vi "PvgeneratorOP300.vi"(8 "errin":errorcluster, 9 "BDD 2":T1, 10 "network":path, 11 "path in":path) -> (0 "sortie d'erreur":errorcluster caption="errout", 1 "network out":path, 2 "tout bon":bool, 3 "Chaîne":string, 5 "chaîne concaténée":string)   [LabVIEW 2020]
uses:
  VG/IS30%.vi
  VG/PN.vi
  <vilib>/Utility/config.llb/NI_LVConfig.lvlib
panel:
  in  "BDD":T1
  out "nombre de remplacements":i32
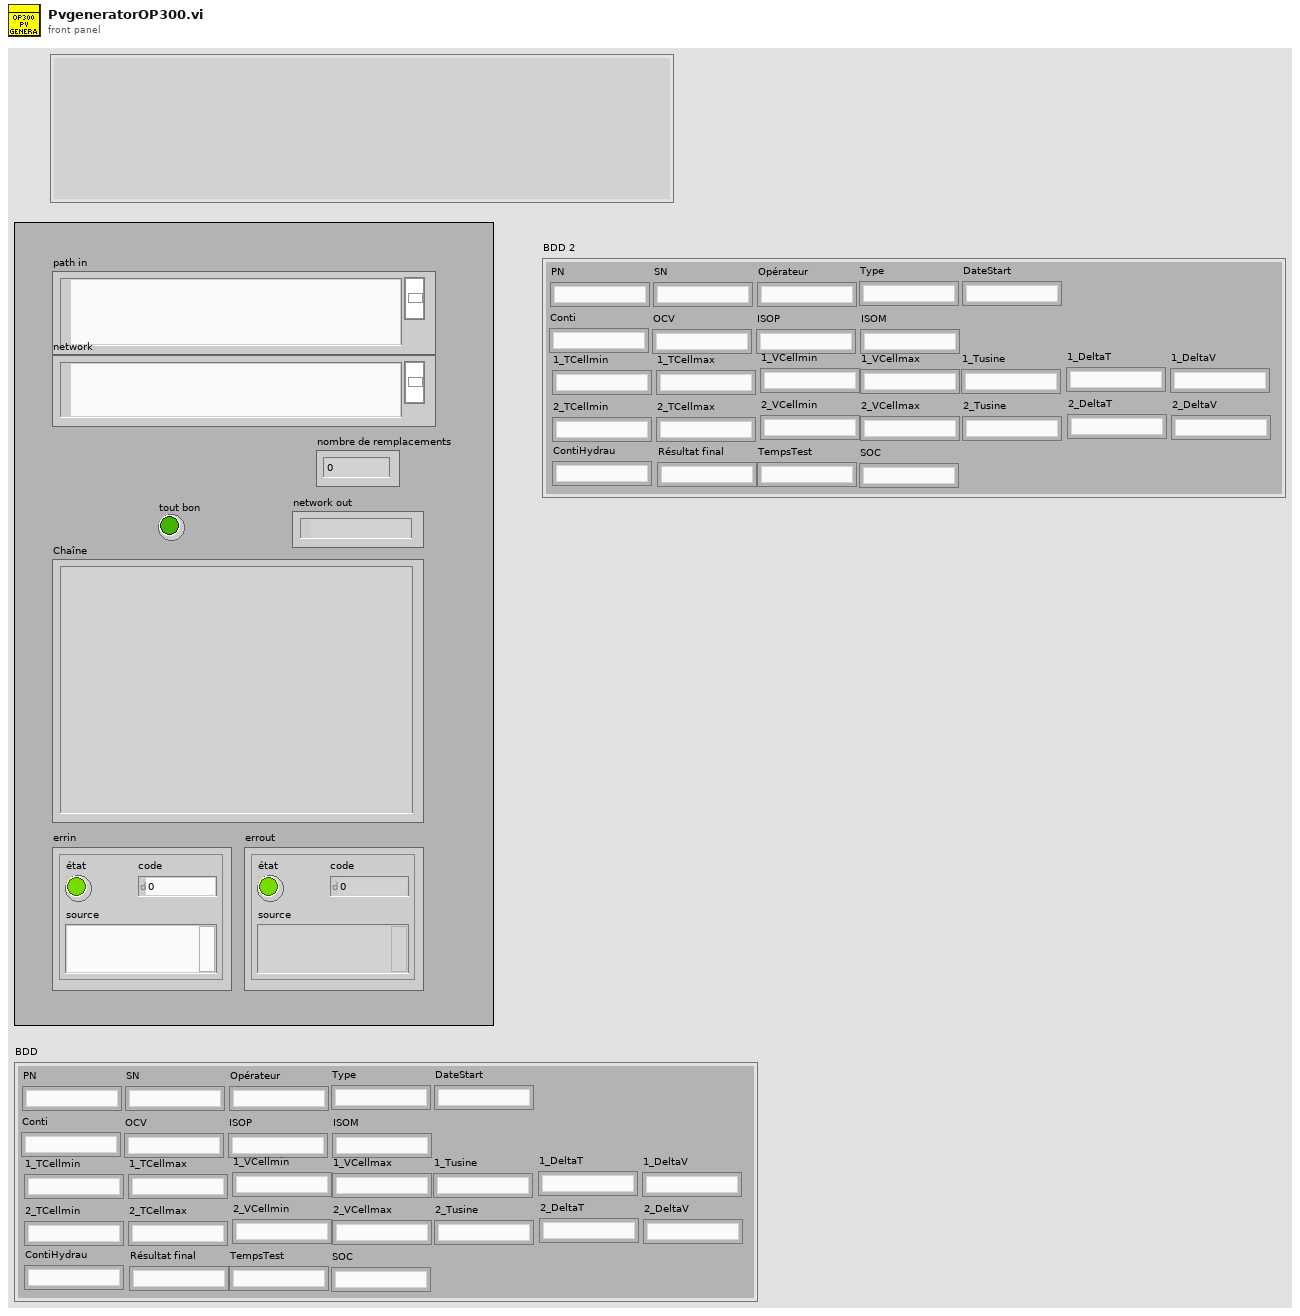
[diagram p1: front panel]
types:
  T1 = cluster{"PN":string, "SN":string, "Opérateur":string, "Type":string, "DateStart":string, "Conti":string, "OCV":string, "ISOP":string, "ISOM":string, "1_TCellmin":string, "1_TCellmax":string, "1_VCellmin":string, "1_VCellmax":string, "1_Tusine":string, "1_DeltaT":string, "1_DeltaV":string, "2_TCellmin":string, "2_TCellmax":string, "2_VCellmin":string, "2_VCellmax":string, "2_Tusine":string, "2_DeltaT":string, "2_DeltaV":string, "ContiHydrau":string, "Résultat final":string, "TempsTest":string, "SOC":string}
  T2 = enum16{"open", "replace", "create", "open or create", "replace or create", "replace or create with confirmation"}
  T3 = typedef "NI_LVConfig.lvlib/Config Data RefNum.ctl" = refnum<k1>
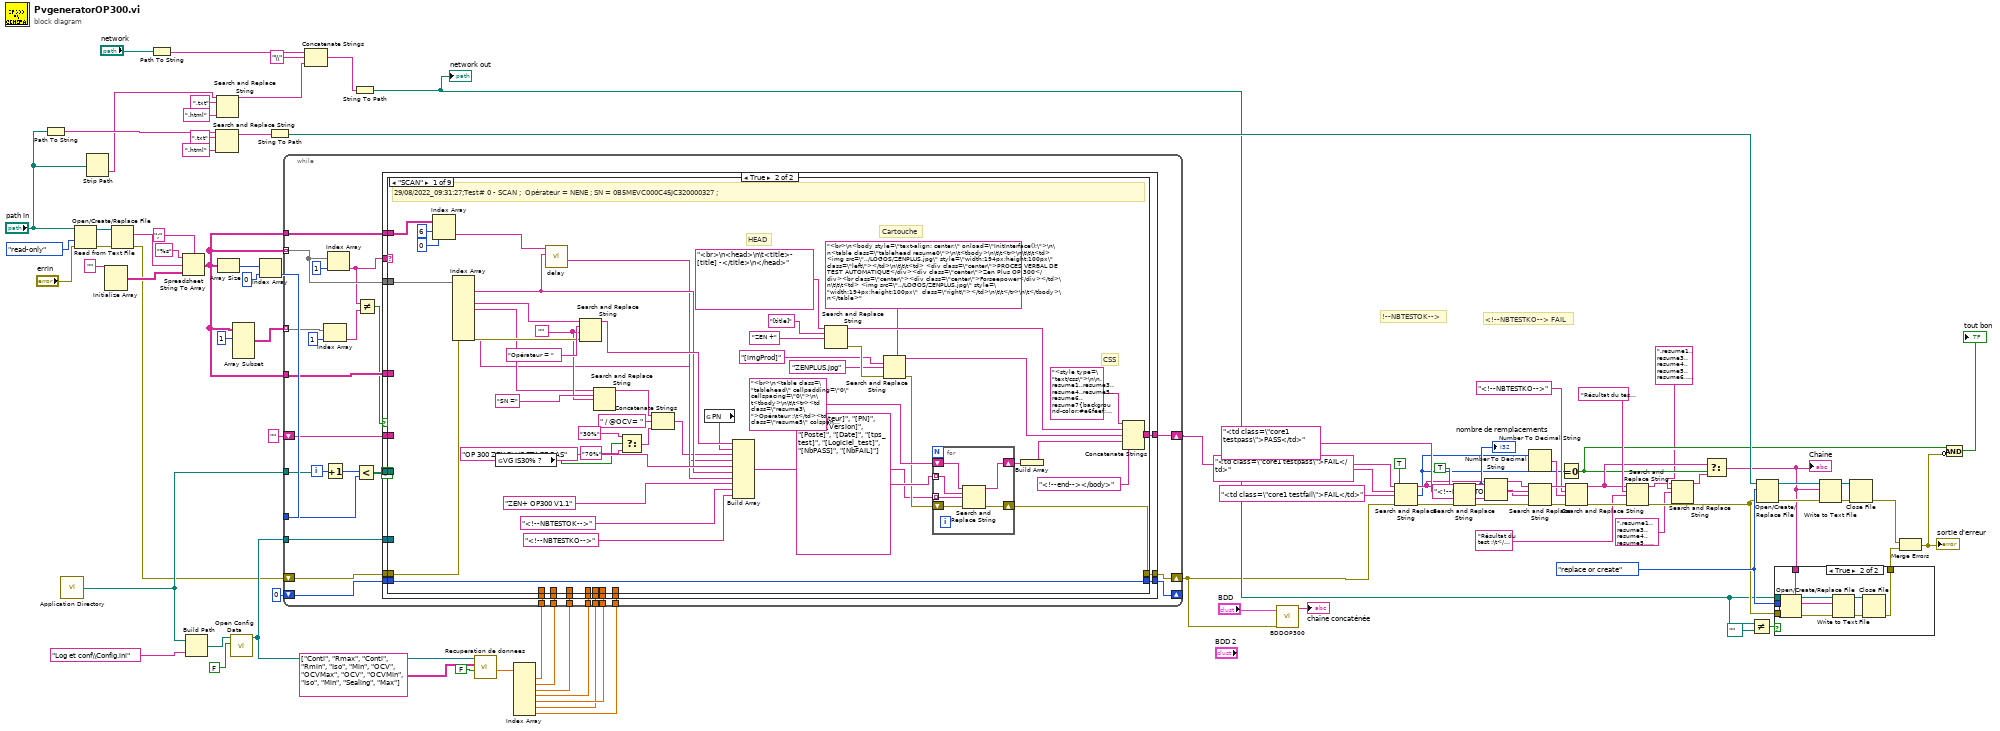
[diagram p0: block diagram]
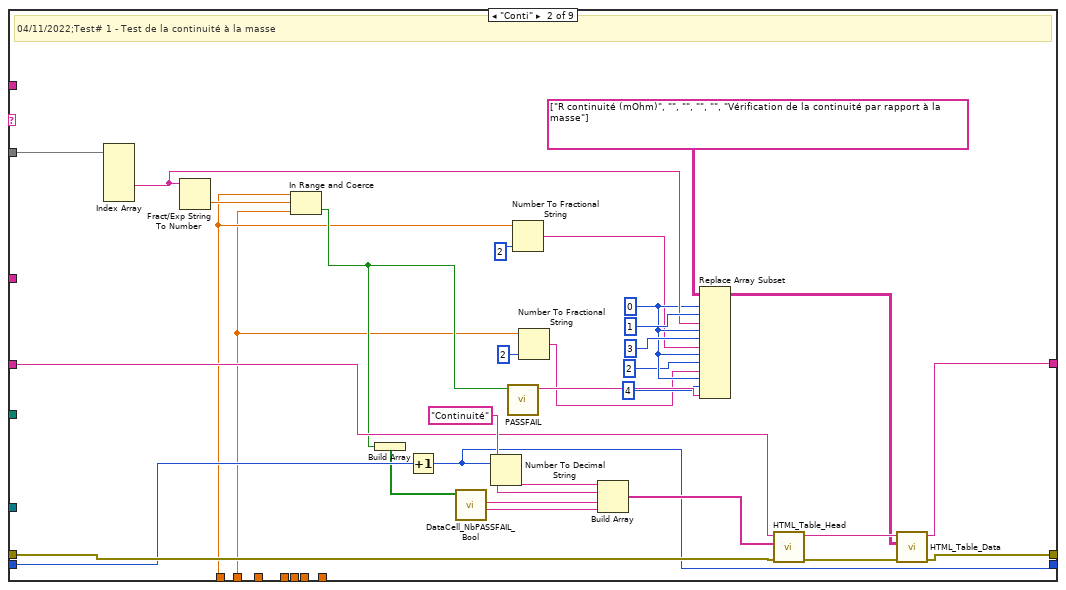
[diagram p3: hidden frame]
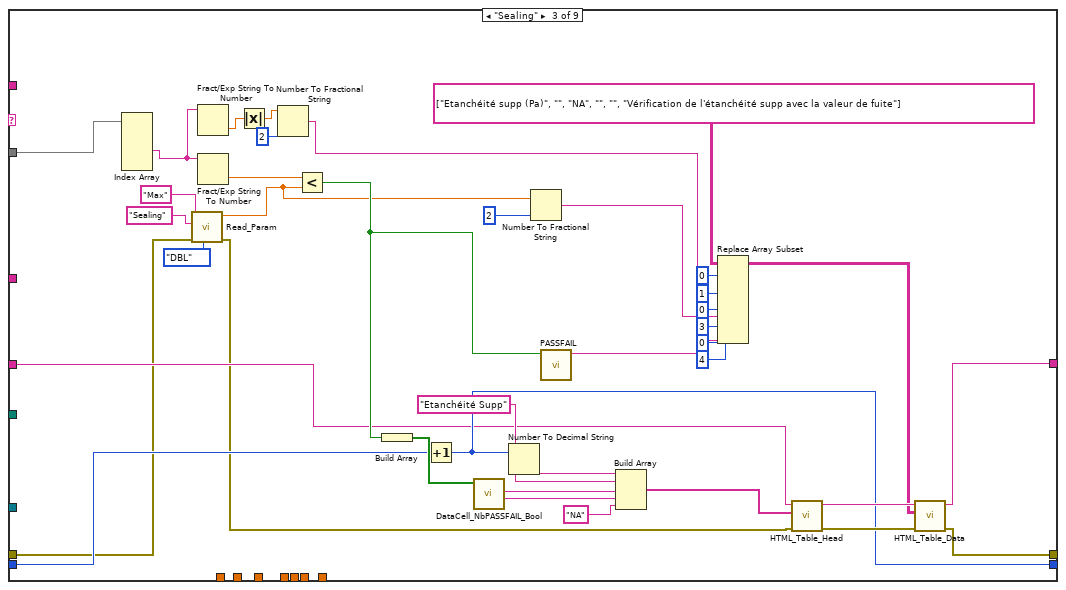
[diagram p4: hidden frame]
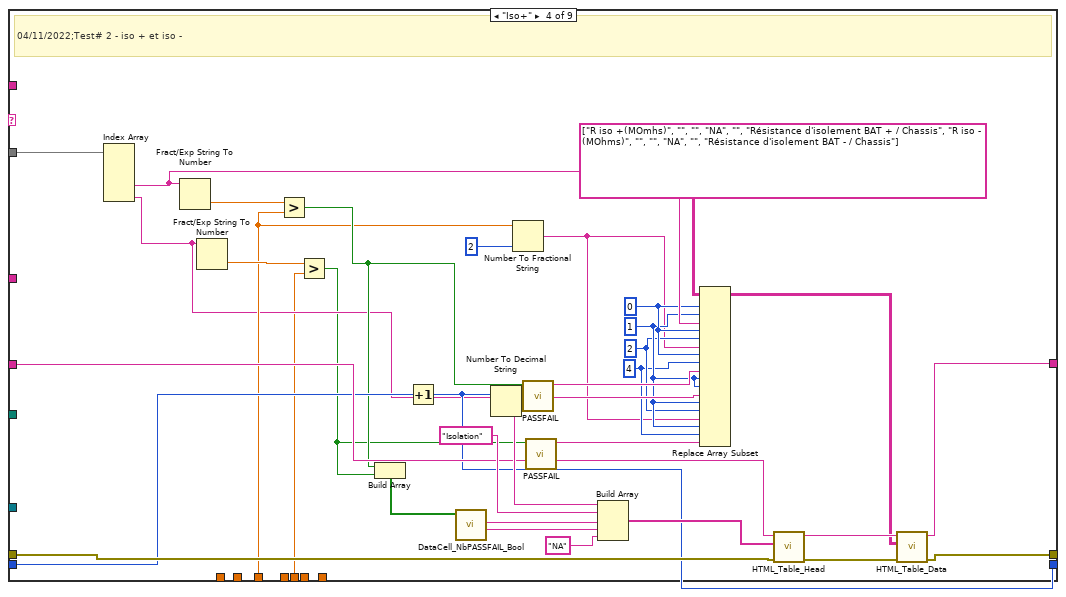
[diagram p5: hidden frame]
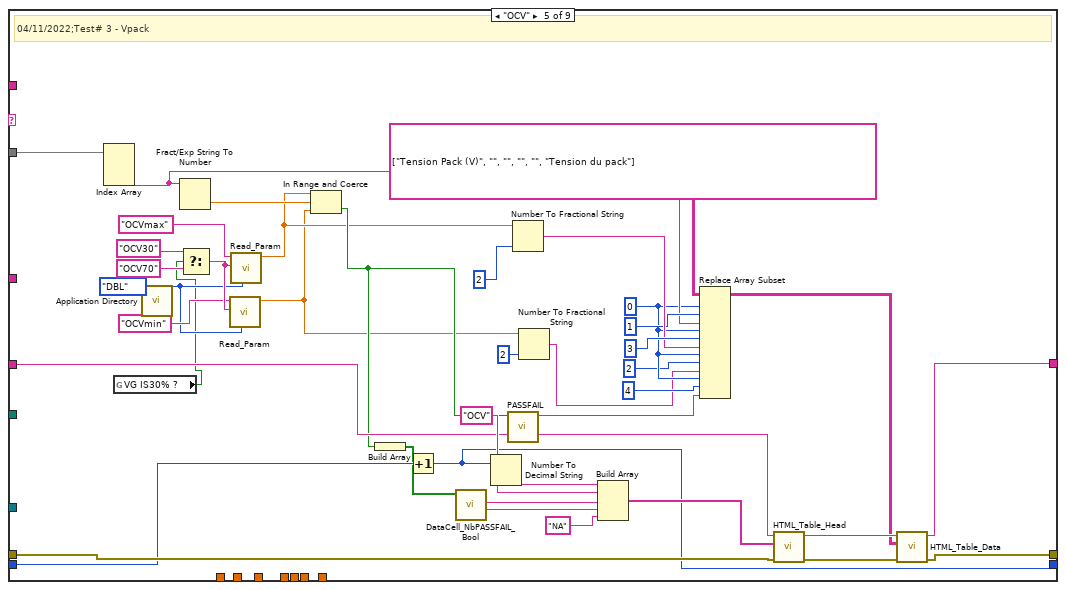
[diagram p6: hidden frame]
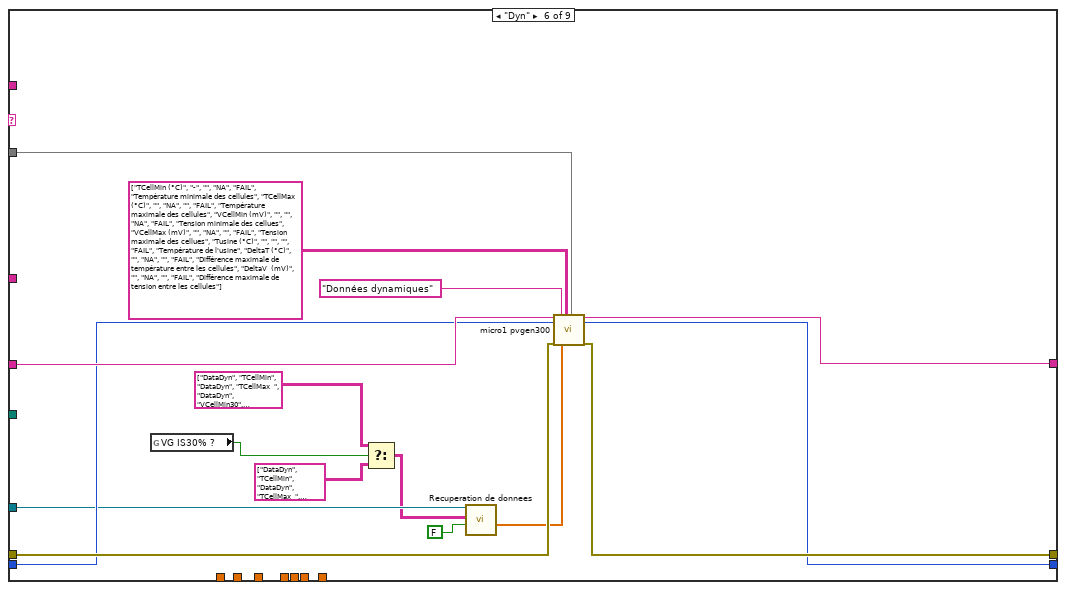
[diagram p7: hidden frame]
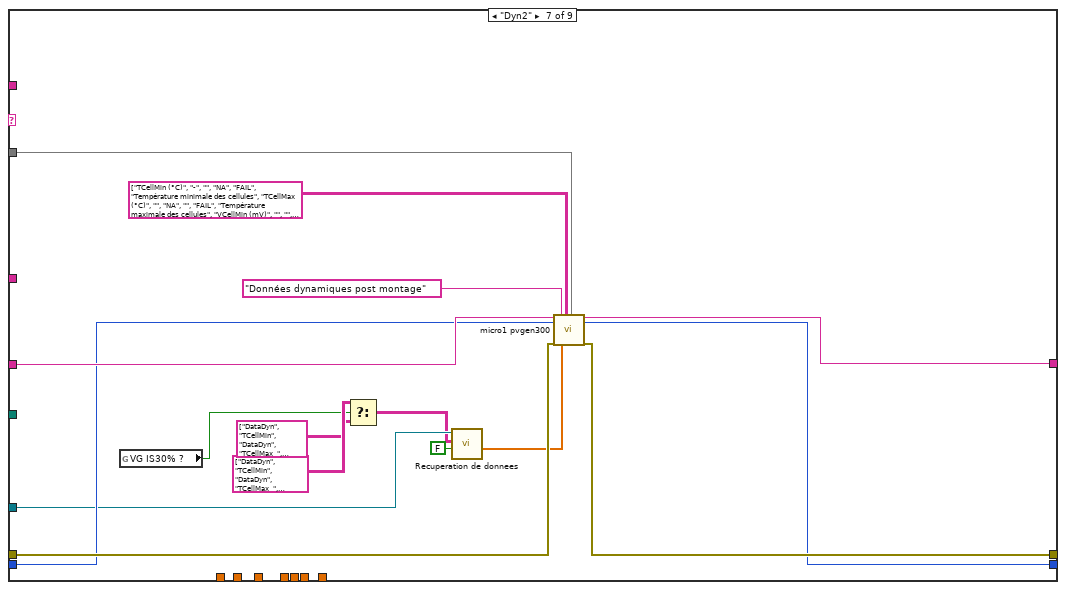
[diagram p8: hidden frame]
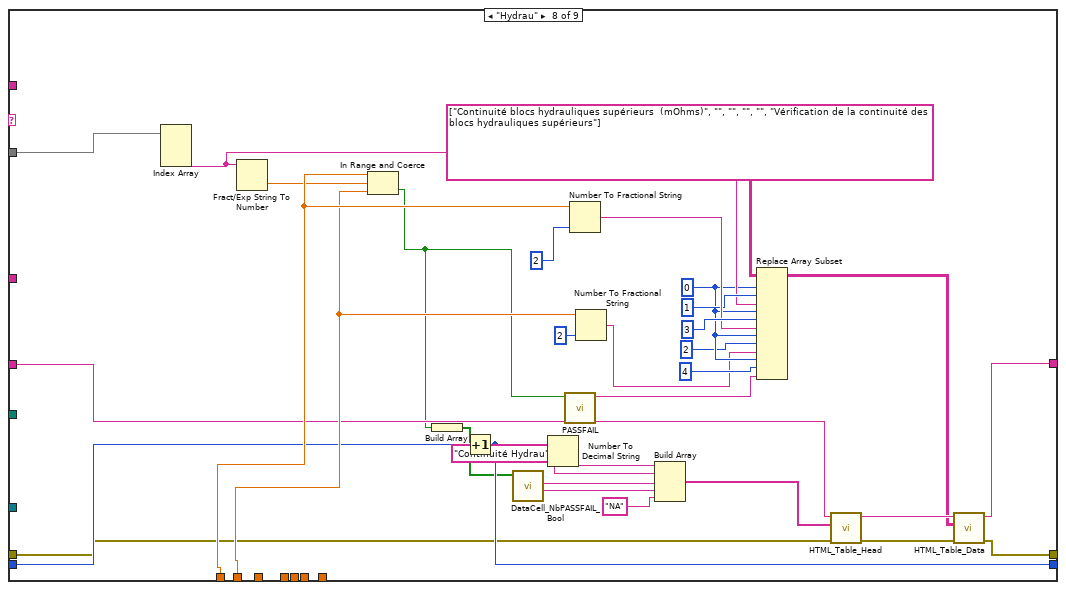
[diagram p9: hidden frame]
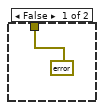
[diagram p11: hidden frame]
diagram:
  w51 = T2."replace or create" ("opération (0 : open)")
  # "<!--NBTESTKO--> FAIL"
  # "!--NBTESTOK-->"
  n1 = Path To String(path="path in") -> (string=w72:string)
  n2 = call <vilib>:"Application Directory.vi"() -> ("Application Directory"=w5:path)
  n3 = Open/Create/Replace File(file path (use dialog)="path in", error in="errin", access (0:read/write)=enum16{"read/write", "read-only", "write-only"}."read-only" ("accès (0 : read/write)")) -> (refnum out=w73:refnum<file>, error out=w89:errorcluster)  [unwired: 3 in, 1 out]
  n4 = Strip Path(path="path in") -> (name=w32:string)  [unwired: 1 out]
  n5 = Initialize Array("") -> (w87:string[][])  [unwired: 2 in]
  n6 = Read from Text File(file (use dialog)=w73, error in=w89) -> (text=w85:string, error out=w4:errorcluster)  [unwired: 2 in, 2 out]
  n7 = Path To String(path="network") -> (string=w31:string)
  n8 = Spreadsheet String To Array(delimiter (Tab)=";" ("séparateur (Tabulation)"), format string="%s" ("chaîne de format"), spreadsheet string=w85, array type (2D Dbl)=w87) -> (array=w11:string[][])
  n9 = Build Path(base path=w5, name or relative path="Log et conf\\Config.ini") -> (appended path=w26:path)
  n10 = Search and Replace String(input string=w72, search string=".txt" ("chaîne recherchée"), replace string=".html" ("chaîne de remplacement (\"\")")) -> (result string=w69:string)  [unwired: 5 in, 3 out]
  n11 = Search and Replace String(input string=w32, search string=".txt" ("chaîne recherchée"), replace string=".html" ("chaîne de remplacement (\"\")")) -> (result string=w29:string)  [unwired: 5 in, 3 out]
  n12 = Array Size(array=w11) -> (size(s)=w83:i32[])
  n13 = call <vilib>:"Open Config Data.vi"("create file if necessary (T)"=FALSE, "configuration file path"=w26) -> ("refnum"=w6:T3)  [unwired: 7 in, 2 out]
  n14 = Array Subset(array=w11, index (row)=1 ("indice")) -> (w9:string[][])  [unwired: 3 in]
  n15 = Index Array(array=w83, index=0 ("indice")) -> (element=w81:i32)
  n16 = String To Path(string=w69) -> (path=w68:path)
  n17 = Concatenate Strings(w31, "\\" ("chaîne"), w29) -> (w28:string)
  n18 = String To Path(string=w28) -> (path=w34:path)
  "network out" <- w34
  n19 = call "Recuperation de donnees.vi"("Est-ce un string?"=FALSE, "Array in"=string[][] [["Conti", "Rmax"], ["Conti", "Rmin"], ["Iso", "Min"], ["OCV", "OCVMax"], ["OCV", "OCVMin"], ["Iso", "Min"], ["Sealing", "Max"]], "Refnum in"=w6) -> ("Array"=w21:dbl[])  [unwired: 7 in, 1 out]
  n20 = Index Array(array=w21) -> (element #1=w20:dbl, element #2=w19:dbl, element #3=w18:dbl, element #4=w17:dbl, element #5=w16:dbl, element #6=w8:dbl, element #7=w7:dbl)  [unwired: 7 in]
  n21 = while {
    tunnel: w81 -> [w117]
    tunnel: w11 -> [w114] mode=indexing
    shift-right: [w113] -> w3
    shift-left: w4 -> [w112]
    shift-right: [w106] -> w67
    shift-left: "" -> [w111]
    shift-right: [w109] -> _
    shift-left: 0 -> [w110]
    tunnel: w11 -> [w108]
    tunnel: w20 -> [w105]
    tunnel: w19 -> [w104]
    tunnel: w11 -> [w103]
    tunnel: w18 -> [w102]
    tunnel: w17 -> [w101]
    tunnel: w16 -> [w100]
    tunnel: w9 -> [w98] mode=indexing
    tunnel: w8 -> [w94]
    tunnel: w7 -> [w93]
    tunnel: w6 -> [w92]
    tunnel: w5 -> [w91]
    i -> [w118]
    stop <- w116 continue-if-true
    n22 = Index Array(array=w98, index=1 ("indice")) -> (element=w97:string)
    n23 = Increment(x=w118) -> (x+1=w107:i32)
    n24 = Index Array(array=w114, index=1 ("indice")) -> (element=w96:string)
    n25 = Less?(x=w107, y=w117) -> (x < y?=w116:bool)
    n26 = Not Equal?(x=w96, y=w97) -> (x != y?=w95:bool)
    n27 = case shown="True" w95 {
      tunnel: w114 -> [_ w140]
      tunnel: [w120 w139] -> w113
      tunnel: w112 -> [w120 w138]
      tunnel: w111 -> [w121 w137]
      tunnel: w110 -> [w119 w136]
      tunnel: [w119 w135] -> w109
      tunnel: w108 -> [_ w134]
      tunnel: [w121 w133] -> w106
      tunnel: w96 -> [_ w132]
      tunnel: w105 -> [_ w122]
      tunnel: w104 -> [_ w131]
      tunnel: w103 -> [_ w130]
      tunnel: w102 -> [_ w129]
      tunnel: w101 -> [_ w128]
      tunnel: w100 -> [_ w127]
      tunnel: w94 -> [_ w126]
      tunnel: w93 -> [_ w125]
      tunnel: w92 -> [_ w124]
      tunnel: w91 -> [_ w123]
      frame False {
      }
      frame True {
        n28 = case shown="\"SCAN\"" w132 {
          tunnel: w138 -> [w185 w218 w233 w290 w330 w354 w370 w397 w406]
          tunnel: w140 -> [w187 w219 w248 w291 w331 w351 w367 w403 _]
          tunnel: [w164 w217 w237 w289 w329 w353 w369 w398 w406] -> w139
          tunnel: w137 -> [_ w216 w234 w288 w328 w350 w366 w396 w404]
          tunnel: w136 -> [w163 w215 w236 w287 w327 w349 w365 w400 w405]
          tunnel: [w163 w214 w235 w286 w326 w348 w364 w399 w405] -> w135
          tunnel: w134 -> [_ _ _ _ _ _ _ _ _]
          tunnel: [w162 w213 w238 w285 w325 w352 w368 w395 w404] -> w133
          tunnel: w131 -> [_ w196 _ _ _ _ _ w401 _]
          tunnel: w130 -> [w144 _ _ _ _ _ _ _ _]
          tunnel: w129 -> [_ _ _ w274 _ _ _ _ _]
          tunnel: w128 -> [_ _ _ _ _ _ _ _ _]
          tunnel: w127 -> [_ _ _ _ _ _ _ _ _]
          tunnel: w126 -> [_ _ _ w265 _ _ _ _ _]
          tunnel: w125 -> [_ _ _ _ _ _ _ _ _]
          tunnel: w124 -> [_ _ _ _ _ w347 w363 _ _]
          tunnel: w123 -> [_ _ _ _ _ _ _ _ _]
          tunnel: w122 -> [_ w197 _ _ _ _ _ w402 _]
          frame "SCAN" {
            w158 = ""
            # "Cartouche"
            # "HEAD"
            # "CSS"
            # "29/08/2022_09:31:27;Test# 0 - SCAN ;  Opérateur = NENE ; SN = 0B5MEVC000C45JC320000327 ;"
            n29 = Index Array(array=w144, index (row)=6, index (col)=0 ("disabled index (col)")) -> (element=w143:string)
            n30 = Index Array(array=w187) -> (element #1=w156:string, element #3=w161:string, element #4=w157:string, element #9=w141:string)  [unwired: 9 in, 5 out]
            n31 = global read "IS30%.vi" "VG IS30% ?"() -> (w149:bool)
            n32 = call "delay.vi"("String"=w156, "String 2"=w143) -> ("Delay calculé"=w147:string)  [unwired: 9 in]
            n33 = Search and Replace String(input string=w161, search string="Opérateur = " ("chaîne recherchée"), replace string=w158, error in=w185) -> (result string=w160:string)  [unwired: 4 in, 3 out]
            n34 = Search and Replace String(input string=w157, search string="SN =" ("chaîne recherchée"), replace string=w158) -> (result string=w154:string)  [unwired: 5 in, 3 out]
            n35 = Select(t="30%" ("y"), s=w149, f="70%" ("y")) -> (s? t:f=w152:string)
            n36 = Concatenate Strings(w154, " / @OCV= " ("chaîne"), w152) -> (w142:string)
            n37 = global read "PN.vi" "PN"() -> (w148:string)
            n38 = Build Array(w160, w148, w142, w141, "OP 300 ZEN PLUS ETAGE BAS" ("chaîne"), w156, w147, "ZEN+ OP300 V1.1" ("chaîne"), "<!--NBTESTOK-->" ("chaîne"), "<!--NBTESTKO-->" ("chaîne")) -> (w165:string[])
            n39 = Search and Replace String(input string="<br>\n<head>\n\t<title>- [title] -</title>\n</head>", search string="[title]" ("chaîne recherchée"), replace string="ZEN +" ("Title")) -> (result string=w181:string, error out=w180:errorcluster)  [unwired: 5 in, 2 out]
            n40 = Search and Replace String(input string="<br>\n<body style=\"text-align: center;\" onload=\"InitInterface();\">\n\n<table class=\"tablehead resume0\">\n\t<tbody>\n\t\t<tr>\n\t\t\t<td> <img src=\"../LOGOS/ZENPLUS.jpg\" style=\"width:194px;height:100px\" class=\"left\"></td>\n\t\t\t<td> <div class=\"center\">PROCES VERBAL DE TEST AUTOMATIQUE</div><div class=\"center\">Zen Plus OP 300</div><br class=\"center\"><div class=\"center\">Forseepower</div></td>\n\t\t\t<td> <img src=\"../LOGOS/ZENPLUS.jpg\" style=\"width:194px;height:100px\"  class=\"right\"></td>\n\t\t</tr>\n\t</tbody>\n</table>", search string="[imgProd]", replace string="ZENPLUS.jpg" ("imgProd"), error in=w180) -> (result string=w178:string, error out=w175:errorcluster)  [unwired: 4 in, 2 out]
            n41 = for {
              shift-right: [w192] -> w174
              shift-left: "<br>\n<table class=\"tablehead\" cellpadding=\"0\" cellspacing=\"0\">\n\t<tbody>\n\t\t<tr><td class=\"resume3\">Opérateur :\t</td><td class=\"resume5\" colspan=\"3\">[Operateur]</td></tr>\n\t\t<tr><td class=\"resume3\">PN : </td><td class=\"resume5\" colspan=\"3\">[PN]</td></tr>\n\t\t<tr><td class=\"resume3\">SN : </td><td class=\"resume5\" colspan=\"3\">[SN]</td></tr>\n\t\t<tr><td class=\"resume3\">Version : </td><td class=\"resume5\" colspan=\"3\">[Version]</td></tr>\n\t\t<tr><td class=\"resume3\">Poste : </td><td class=\"resume5\" colspan=\"3\">[Poste]</td></tr>\t\t\n\t\t<tr><td class=\"resume3\">Date du test : </td><td class=\"resume5\" colspan=\"3\">[Date]</td></tr>\n\t\t<tr><td class=\"resume3\">Temps de test : </td><td class=\"resume5\" colspan=\"3\">[tps_test]</td></tr>\n\t\t<tr><td class=\"resume3\">Logiciel de test :\t</td><td class=\"resume5\" colspan=\"3\">[Logiciel_test]</td></tr>\n\t\t<tr><td class=\"resume3\">Résultat du test :\t</td><td class=\"resume5\" colspan=\"3\"><div><span style=\"float:left\" id=\"result\"><font size = \"5pt\" color=\"green\"><b>CONFORME</b></font><b><font size = \"5pt\"> ( </font><font size = \"5pt\" color=\"green\">[NbPASS] PASS </font>  <font size = \"5pt\"> / </font><font size = \"5pt\" color=\"red\">[NbFAIL] FAIL</font> <font size = \"5pt\"> ) </font></b></span></div></td></tr>\n\t</tbody>\n</table>" -> [w193]
              tunnel: string[] ["[Operateur]", "[PN]", "[SN]", "[Version]", "[Poste]", "[Date]", "[tps_test]", "[Logiciel_test]", "[NbPASS]", "[NbFAIL]"] -> [w189] mode=indexing
              tunnel: w165 -> [w188] mode=indexing
              shift-right: [w190] -> w164
              shift-left: w175 -> [w191]
              n42 = Search and Replace String(input string=w193, search string=w189, replace string=w188, error in=w191) -> (result string=w192:string, error out=w190:errorcluster)  [unwired: 4 in, 2 out]
            }
            n43 = Build Array(w174) -> (w173:string[])
            n44 = Concatenate Strings("<style type=\"text/css\">\n\n.resume1,.resume3,.resume4,.resume5,.resume6,.resume7{background-color:#e6feef;padding:7px;border:1px solid black;}\n.resume0{border:1px solid black;background-color:#e6feef;font-weight: bold;padding:0px;text-align: center;}\n.resume1{width:350px;text-align:right;font-weight:bold;}\n.resume3{width:350px;text-align:right;border-top:0px solid black;font-weight:bold;}\n.resume4{border-left:0px solid black;width:290px;}\n.resume5{width:290px;border-left:0px solid black;border-top:0px solid black;}\n.resume6{border-left:0px solid black;width:60px;}\n.resume7{border-left:0px solid black;border-top:0px solid black;width:60px;}\n.title1{text-align: left;background-color:#e6f4fe;padding:10px;border:1px solid #101010;}\n.title2{width: 30px;text-align: center;background-color:#e6f4fe;padding:1px;border:1px solid #101010;border-left:0px solid black;font-weight: bold;}\n.title2 a:link{text-decoration:none;}\n.entete0,.entete1,.entete2,.time2{text-align: center;background-color:#feeec9;padding:7px;border:1px solid black;font-weight: bold;}\n.entete0{width:45px;border-right:0px solid black;}\n.entete1{width:505px;}\n.entete2{width:95px;border-right:0px solid black;}\n.time2{border-left:0px solid black;width:145px;font-size:11px;}\n.core0,.core1,.core2,.core3,.core4,.time{text-align: center;background-color:#fafed3;padding:7px;border:1px solid black;}\n.core0, .core1,.core3,.core4{width:95px;border-top:0px solid black;border-right:0px solid black;}\n.core0{width:45px;}\n.core2{border-top:0px solid black;width:505px;}\n.core3{width:200px;}\n.core4{width:300px;}\n.time{width:145px;border-top:0px solid black;border-left:0px solid black;font-size:11px;}\n.false .core0,.false .core1,.false .core2,.false .core3,.false .core4,.false .time{background-color:#f4f4f4;}\n.false .entete0,.false .entete1,.false .entete2,.false .time2{background-color:#dadada;}\n.false .title1,.false .title2,.false .resultentete .testpass,.false .resultentete .testfail,.false .resultentete .testtime{background-color:#c5cac9;color: blue;}\n.false .title2 a:link{text-decoration:none;color: blue;}\n.comment1,.comment2,.time3{width: 890px;background-color:#e9e8e9;padding:7px;border:1px solid black;border-top:0px solid black;text-align:left;}\n.comment2{border-right:0px solid black;width: 45px;text-align: center;}\n.time3{width: 145px;border-left:0px solid black;font-size:11px;}\n.fixe1{background: -moz-linear-gradient(center top , #101010 10%, #555555 80%) repeat scroll 0 0 transparent;background: -webkit-gradient(linear, left top, left bottom, from(#101010), to(#555555));border:2px solid orange;position : fixed;margin-top:20px;display:none;overflow-y:scroll;max-height:350px;text-shadow: 0px 0px 0 #333333;text-align:left;font-size:10px;padding:10px;margin-left:-162px;border-radius: 15px 15px 15px 15px;}\n.menufixe, .menufixelock{background: -moz-linear-gradient(center top , #101010 80%, transparent 20%) repeat scroll 0 0 transparent;background: -webkit-gradient(linear, left top, left bottom, from(#101010), color-stop(0.65, #101010), to(transparent)) repeat scroll 0 0 transparent;margin: -52px 0px 0px -9px;width:100%;position:fixed;height:55px;-moz-transition: margin 1s;-webkit-transition: margin 1s;}\n.menufixelock, .menufixe:hover{margin: -9px 0px 0px -9px;}\n.lockmenu, .separation,.separationmenu{text-align:center;background: -moz-linear-gradient(center top , #555555 10%, #111111 80%) repeat scroll 0 0 transparent;background: -webkit-gradient(linear, left top, left bottom, from(#555555), to(#111111));border: 1px solid white;border-radius: 10px 10px 10px 10px;box-shadow: 0 -1px 1px #555555 inset;color: #999999;font-weight: bold;width: 100px;padding: 2px;text-decoration: none;}\n.tablehead{width: 1000px;font-family: Verdana;font-size: 12px;margin-left: auto;margin-right: auto;}\n.tablenull{font-family: Verdana;font-size: 11px;margin-left: auto;margin-right: auto;}\n.separationmenu:hover div{display: inline;}\n.lockmenu:hover, .separation:hover,.separationmenu:hover{border: 1px solid orange;cursor:pointer;}\n.lockmenu:hover{border: 1px solid red;cursor:pointer;}\n.separationright{padding:10px;}\ndiv a:link{text-decoration:none;color:#cbcbcb;}\ndiv a:hover{text-decoration:underline;color:#cbcbcb;}\nspan a:link{text-decoration:none;color:#cbcbcb;}\nspan a:hover{text-decoration:none;color:#cbcbcb;}\n.false{color: blue;}\n.testpass{color: green;font-weight: bold;}\n.testfail{color: red;font-weight: bold;}\n.testtime{color: blue;font-weight: bold;}\n.resultentete{font-weight: bold;font-size: 11px;min-width: 200px;text-align:right;}\n.infohard{border: 1px solid black;background-color: white;text-align: center;width: 16px;height: 16px;border-radius: 5px;font-weight: bold;box-shadow: 0 -1px 2px #555555 inset;}\n.infohard:hover{background-color:#feeec9;cursor:pointer;}\n.footerhard{padding-top:30px;}\n.confighard{font-size:10px;width:110px;}\n.circlemain{margin-left:auto;margin-right:auto;}\n.circletext,.circleform{padding-top: 3px;text-align:center;font-size: 10px;width:200px;}\n.circleform{padding-bottom: 3px;padding-top: 1px;}\n.circle{border: 1px solid black;border-collapse: collapse;border-radius: 15px;box-shadow: 1px 1px 0 #505050;height: 15px;width: 15px;display:inline-block;}\n.bookmarkon, .bookmarkoff{background-color: yellow;border: 1px solid black;border-collapse: collapse;border-radius: 10px 10px 10px 10px;box-shadow: 1px 1px 0 #505050;height: 12px;width: 12px;position: absolute;margin-left:22px;cursor: help;}\n.bookmarkoff{background-color: transparent;border: 1px solid #CECECE;box-shadow: none;cursor: copy;}\n.false .bookmarkoff{background-color: transparent;border: 1px solid #E6E1E1;box-shadow: none;cursor: copy;}\n.bookmarkmaster{height: 15px;margin-right: 12px;width: 60px;}\n.bookmarkmaster:hover .bookmarkprev,.bookmarkmaster:hover .bookmarksuiv{display:block;}\n.bookmarkprev, .bookmarksuiv {cursor: pointer;font-size: 25px;font-weight: bold;margin-top: -10px;position: absolute;display:none;}\n.bookmarkprev{margin-left: 2px;}\n.bookmarksuiv{margin-left: 43px;}\n.plus, .moins{background-color: #F4F4F4;border: 1px solid #848484;border-radius: 20px;color: #848484;font-family: arial;font-size: 16px;font-weight: bold;height: 20px;margin-left: 4px;text-align: center;width: 20px;}\n.moins{font-size: 15px;}\n.plus:hover, .moins:hover{background-color: #DADADA;border: 1px solid black;color: black;cursor:pointer;}\n.backtothetop {position: fixed; right: 50%; margin-right: -555px; bottom: 10px; font-size: 35px; font-weight: bold; border: 1px solid #7D7B91; width: 40px; height: 40px; line-height:52px; text-align: center;border-radius: 8px; opacity: 0.25; background-color: #F5F5F5; color:#7D7B91;}\n.backtothetop:hover {opacity: 1; cursor:pointer;}\n.libversion {font-size: 8px;font-weight: normal;padding-right: 10px;text-align: right;}\n.lockmenu {width: 18px;font-size: 12px;}\n.left {display: block; margin-left: 1px;margin-right: auto;}\n.right {display: block; margin-right: 1px;margin-left: auto;}\n.center {display: block; margin-left: auto;margin-right: auto;}\n\n</style>", w181, w178, w173, "<!--end--></body>") -> (w162:string)
          }
          frame "Conti" {
            w201 = 0 ("index (row)")
            # "04/11/2022;Test# 1 - Test de la continuité à la masse"
            n45 = Index Array(array=w219) -> (element #3=w205:string)  [unwired: 5 in, 4 out]
            n46 = Fract/Exp String To Number(string=w205) -> (number=w204:dbl)  [unwired: 3 in, 1 out]
            n47 = In Range and Coerce(upper limit=w197, x=w204, lower limit=w196) -> (In Range?=w199:bool)  [unwired: 1 out]
            n48 = Build Array(w199) -> (w211:bool[])
            n49 = Increment(x=w215) -> (x+1=w214:i32)
            n50 = call "DataCell_NbPASSFAIL_Bool.vi"("Tableau en entrée"=w211) -> ("Chaîne"=w209:string, "Chaîne 2"=w210:string)  [unwired: 8 in, 1 out]
            n51 = Number To Decimal String(number=w214) -> (decimal integer string=w221:string)  [unwired: 1 in]
            n52 = call <userlib>:"PASSFAIL.vi"("E"=w199) -> ("S"=w203:string)  [unwired: 10 in]
            n53 = Number To Fractional String(number=w197, precision (6)=i16 2) -> (F-format string=w194:string)  [unwired: 2 in]
            n54 = Number To Fractional String(number=w196, precision (6)=i16 2) -> (F-format string=w195:string)  [unwired: 2 in]
            n55 = Build Array(w221, "Continuité" ("élément"), w210, w209) -> (w224:string[])
            n56 = Replace Array Subset(array=string[][] [["R continuité (mOhm)", "", "", "", "", "Vérification de la continuité par rapport à la masse"]] ("Tableau"), new element #1=w205, index (row) #1=w201, index (col) #1=1 ("disabled index (col)"), new element #2=w194, index (row) #2=w201, index (col) #2=3 ("disabled index (col)"), new element #3=w195, index (row) #3=w201, index (col) #3=2 ("disabled index (col)"), new element #4=w203, index (row) #4=w201, index (col) #4=4 ("disabled index (col)")) -> (w212:string[][])
            n57 = call "HTML_Table_Head.vi"("entrée d'erreur (pas d'erreur)"=w218, "Tableau"=w224, "chaîne en entrée"=w216) -> ("sortie d'erreur"=w223:errorcluster, "result string"=w222:string)  [unwired: 7 in]
            n58 = call "HTML_Table_Data.vi"("entrée d'erreur (pas d'erreur)"=w223, "Tableau"=w212, "chaîne en entrée"=w222) -> ("sortie d'erreur"=w217:errorcluster, "result string"=w213:string)  [unwired: 7 in]
          }
          frame "Sealing" {
            n59 = Index Array(array=w248) -> (element #3=w230:string)  [unwired: 5 in, 4 out]
            n60 = call <userlib>:"Read_Param.vi"("Énum"=enum16{"STR", "DBL", "U32", "chemin"}."DBL", "errin"=w233, "section"="Sealing", "key"="Max") -> ("error out"=w232:errorcluster, "dbl"=w245:dbl)  [unwired: 3 in, 3 out]
            n61 = Fract/Exp String To Number(string=w230) -> (number=w229:dbl)  [unwired: 3 in, 1 out]
            n62 = Fract/Exp String To Number(string=w230) -> (number=w252:dbl)  [unwired: 3 in, 1 out]
            n63 = Absolute Value(x=w229) -> (abs(x)=w228:dbl)
            n64 = Number To Fractional String(number=w228, precision (6)=i16 2 ("précision (6)")) -> (F-format string=w227:string)  [unwired: 2 in]
            n65 = Less?(x=w252, y=w245) -> (x < y?=w251:bool)
            n66 = Build Array(w251) -> (w256:bool[])
            n67 = Increment(x=w236) -> (x+1=w235:i32)
            n68 = call "DataCell_NbPASSFAIL_Bool.vi"("Tableau en entrée"=w256) -> ("Chaîne"=w254:string, "Chaîne 2"=w255:string)  [unwired: 8 in, 1 out]
            n69 = Number To Decimal String(number=w235) -> (decimal integer string=w260:string)  [unwired: 1 in]
            n70 = Number To Fractional String(number=w245, precision (6)=i16 2) -> (F-format string=w249:string)  [unwired: 2 in]
            n71 = call <userlib>:"PASSFAIL.vi"("E"=w251) -> ("S"=w250:string)  [unwired: 10 in]
            n72 = Build Array(w260, "Etanchéité Supp" ("élément"), w255, w254, "NA" ("élément")) -> (w263:string[])
            n73 = Replace Array Subset(array=string[][] [["Etanchéité supp (Pa)", "", "NA", "", "", "Vérification de l'étanchéité supp avec la valeur de fuite"]] ("Tableau"), new element #1=w227, index (row) #1=0 ("indice (ligne)"), index (col) #1=1 ("indice désactivé (col)"), new element #2=w249, index (row) #2=0 ("indice (ligne)"), index (col) #2=3 ("indice désactivé (col)"), new element #3=w250, index (row) #3=0 ("indice (ligne)"), index (col) #3=4 ("indice désactivé (col)")) -> (w257:string[][])
            n74 = call "HTML_Table_Head.vi"("entrée d'erreur (pas d'erreur)"=w232, "Tableau"=w263, "chaîne en entrée"=w234) -> ("sortie d'erreur"=w262:errorcluster, "result string"=w261:string)  [unwired: 7 in]
            n75 = call "HTML_Table_Data.vi"("entrée d'erreur (pas d'erreur)"=w262, "Tableau"=w257, "chaîne en entrée"=w261) -> ("sortie d'erreur"=w237:errorcluster, "result string"=w238:string)  [unwired: 7 in]
          }
          frame "Iso+" {
            w269 = 4 ("disabled index (col)")
            w270 = 2 ("disabled index (col)")
            w271 = 1 ("disabled index (col)")
            w278 = 0 ("index (row)")
            # "04/11/2022;Test# 2 - iso + et iso -"
            n76 = Index Array(array=w291) -> (element #3=w279:string, element #5=w272:string)  [unwired: 5 in, 3 out]
            n77 = Fract/Exp String To Number(string=w279) -> (number=w277:dbl)  [unwired: 3 in, 1 out]
            n78 = Fract/Exp String To Number(string=w272) -> (number=w275:dbl)  [unwired: 3 in, 1 out]
            n79 = Greater?(x=w277, y=w274) -> (0:w276:bool)
            n80 = Greater?(x=w275, y=w265) -> (0:w267:bool)
            n81 = Build Array(w276, w267) -> (w283:bool[])
            n82 = Increment(x=w287) -> (x+1=w286:i32)
            n83 = call "DataCell_NbPASSFAIL_Bool.vi"("Tableau en entrée"=w283) -> ("Chaîne"=w281:string, "Chaîne 2"=w282:string)  [unwired: 8 in, 1 out]
            n84 = Number To Decimal String(number=w286) -> (decimal integer string=w294:string)  [unwired: 1 in]
            n85 = Number To Fractional String(number=w274, precision (6)=i16 2) -> (F-format string=w268:string)  [unwired: 2 in]
            n86 = call <userlib>:"PASSFAIL.vi"("E"=w276) -> ("S"=w273:string)  [unwired: 10 in]
            n87 = call <userlib>:"PASSFAIL.vi"("E"=w267) -> ("S"=w266:string)  [unwired: 10 in]
            n88 = Build Array(w294, "Isolation" ("élément"), w282, w281, "NA" ("élément")) -> (w297:string[])
            n89 = Replace Array Subset(array=string[][] [["R iso +(MOmhs)", "", "", "NA", "", "Résistance d'isolement BAT + / Chassis"], ["R iso - (MOhms)", "", "", "NA", "", "Résistance d'isolement BAT - / Chassis"]] ("Tableau"), new element #1=w279, index (row) #1=w278, index (col) #1=w271, new element #2=w268, index (row) #2=w278, index (col) #2=w270, new element #3=w273, index (row) #3=w278, index (col) #3=w269, new element #4=w272, index (row) #4=w271, index (col) #4=w271, new element #5=w268, index (row) #5=w271, index (col) #5=w270, new element #6=w266, index (row) #6=w271, index (col) #6=w269) -> (w284:string[][])
            n90 = call "HTML_Table_Head.vi"("entrée d'erreur (pas d'erreur)"=w290, "Tableau"=w297, "chaîne en entrée"=w288) -> ("sortie d'erreur"=w296:errorcluster, "result string"=w295:string)  [unwired: 7 in]
            n91 = call "HTML_Table_Data.vi"("entrée d'erreur (pas d'erreur)"=w296, "Tableau"=w284, "chaîne en entrée"=w295) -> ("sortie d'erreur"=w289:errorcluster, "result string"=w285:string)  [unwired: 7 in]
          }
          frame "OCV" {
            w302 = enum16{"STR", "DBL", "U32"}."DBL" ("Énum")
            w312 = 0 ("index (row)")
            # "04/11/2022;Test# 3 - Vpack"
            n92 = Index Array(array=w331) -> (element #3=w316:string)  [unwired: 3 in, 2 out]
            n93 = global read "IS30%.vi" "VG IS30% ?"() -> (w299:bool)
            n94 = call <vilib>:"Application Directory.vi"() -> ()  [unwired: 1 out]
            n95 = Fract/Exp String To Number(string=w316) -> (number=w315:dbl)  [unwired: 3 in, 1 out]
            n96 = Select(t="OCV30" ("section"), s=w299, f="OCV70" ("section")) -> (s? t:f=w305:string)
            n97 = call <userlib>:"Read_Param.vi"("Énum"=w302, "section"=w305, "key"="OCVmin") -> ("dbl"=w300:dbl)  [unwired: 4 in, 4 out]
            n98 = call <userlib>:"Read_Param.vi"("Énum"=w302, "section"=w305, "key"="OCVmax") -> ("dbl"=w301:dbl)  [unwired: 4 in, 4 out]
            n99 = In Range and Coerce(upper limit=w301, x=w315, lower limit=w300) -> (In Range?=w310:bool)  [unwired: 1 out]
            n100 = Build Array(w310) -> (w323:bool[])
            n101 = Increment(x=w327) -> (x+1=w326:i32)
            n102 = call "DataCell_NbPASSFAIL_Bool.vi"("Tableau en entrée"=w323) -> ("Chaîne"=w321:string, "Chaîne 2"=w322:string)  [unwired: 8 in, 1 out]
            n103 = Number To Decimal String(number=w326) -> (decimal integer string=w334:string)  [unwired: 1 in]
            n104 = call <userlib>:"PASSFAIL.vi"("E"=w310) -> ("S"=w314:string)  [unwired: 10 in]
            n105 = Number To Fractional String(number=w301, precision (6)=i16 2) -> (F-format string=w319:string)  [unwired: 2 in]
            n106 = Number To Fractional String(number=w300, precision (6)=i16 2) -> (F-format string=w308:string)  [unwired: 2 in]
            n107 = Build Array(w334, "OCV" ("élément"), w322, w321, "NA" ("élément")) -> (w337:string[])
            n108 = Replace Array Subset(array=string[][] [["Tension Pack (V)", "", "", "", "", "Tension du pack"]] ("Tableau"), new element #1=w316, index (row) #1=w312, index (col) #1=1 ("disabled index (col)"), new element #2=w319, index (row) #2=w312, index (col) #2=3 ("disabled index (col)"), new element #3=w308, index (row) #3=w312, index (col) #3=2 ("disabled index (col)"), new element #4=w314, index (row) #4=w312, index (col) #4=4 ("disabled index (col)")) -> (w324:string[][])
            n109 = call "HTML_Table_Head.vi"("entrée d'erreur (pas d'erreur)"=w330, "Tableau"=w337, "chaîne en entrée"=w328) -> ("sortie d'erreur"=w336:errorcluster, "result string"=w335:string)  [unwired: 7 in]
            n110 = call "HTML_Table_Data.vi"("entrée d'erreur (pas d'erreur)"=w336, "Tableau"=w324, "chaîne en entrée"=w335) -> ("sortie d'erreur"=w329:errorcluster, "result string"=w325:string)  [unwired: 7 in]
          }
          frame "Dyn" {
            n111 = global read "IS30%.vi" "VG IS30% ?"() -> (w340:bool)
            n112 = Select(t=string[][] [["DataDyn", "TCellMin"], ["DataDyn", "TCellMax  "], ["DataDyn", "VCellMin30"], ["DataDyn", "VCellMax30"], ["DataDyn", "TusineMax"], ["DataDyn", "TusineMin"], ["DataDyn", "DeltaT "], ["DataDyn", "DeltaV "]], s=w340, f=string[][] [["DataDyn", "TCellMin"], ["DataDyn", "TCellMax  "], ["DataDyn", "VCellMin70 "], ["DataDyn", "VCellMax70"], ["DataDyn", "TusineMax"], ["DataDyn", "TusineMin"], ["DataDyn", "DeltaT "], ["DataDyn", "DeltaV "]]) -> (s? t:f=w341:string[][])
            n113 = call "Recuperation de donnees.vi"("Est-ce un string?"=FALSE, "Array in"=w341, "Refnum in"=w347) -> ("Array"=w343:dbl[])  [unwired: 7 in, 1 out]
            n114 = call "micro1 pvgen300.vi"("FluxStrIn"=w350, "Numin"=w349, "errin"=w354, "testlabel"="Données dynamiques", "Data limit"=w343, "tab ref"=string[][] [["TCellMin (°C)", "-", "", "NA", "FAIL", "Température minimale des cellules"], ["TCellMax (°C)", "", "NA", "", "FAIL", "Température maximale des cellules"], ["VCellMin (mV)", "", "", "NA", "FAIL", "Tension minimale des cellues"], ["VCellMax (mV)", "", "NA", "", "FAIL", "Tension maximale des cellues"], ["Tusine (°C)", "", "", "", "FAIL", "Température de l'usine"], ["DeltaT (°C)", "", "NA", "", "FAIL", "Différence maximale de température entre les cellules"], ["DeltaV  (mV)", "", "NA", "", "FAIL", "Différence maximale de tension entre les cellules"]] ("Tableau"), "ligne à traiter"=w351) -> ("result string"=w352:string, "Numout"=w348:i32, "errout"=w353:errorcluster)  [unwired: 10 in]
          }
          frame "Dyn2" {
            n115 = global read "IS30%.vi" "VG IS30% ?"() -> (w355:bool)
            n116 = Select(t=string[][] [["DataDyn", "TCellMin"], ["DataDyn", "TCellMax  "], ["DataDyn", "VCellMin30"], ["DataDyn", "VCellMax30"], ["DataDyn", "TusineMax"], ["DataDyn", "TusineMin"], ["DataDyn", "DeltaT "], ["DataDyn", "DeltaV "]], s=w355, f=string[][] [["DataDyn", "TCellMin"], ["DataDyn", "TCellMax  "], ["DataDyn", "VCellMin70 "], ["DataDyn", "VCellMax70"], ["DataDyn", "TusineMax"], ["DataDyn", "TusineMin"], ["DataDyn", "DeltaT "], ["DataDyn", "DeltaV "]]) -> (s? t:f=w357:string[][])
            n117 = call "Recuperation de donnees.vi"("Est-ce un string?"=FALSE, "Array in"=w357, "Refnum in"=w363) -> ("Array"=w356:dbl[])  [unwired: 7 in, 1 out]
            n118 = call "micro1 pvgen300.vi"("FluxStrIn"=w366, "Numin"=w365, "errin"=w370, "testlabel"="Données dynamiques post montage", "Data limit"=w356, "tab ref"=string[][] [["TCellMin (°C)", "-", "", "NA", "FAIL", "Température minimale des cellules"], ["TCellMax (°C)", "", "NA", "", "FAIL", "Température maximale des cellules"], ["VCellMin (mV)", "", "", "NA", "FAIL", "Tension minimale des cellues"], ["VCellMax (mV)", "", "NA", "", "FAIL", "Tension maximale des cellues"], ["Tusine (°C)", "", "", "", "FAIL", "Température de l'usine"], ["DeltaT (°C)", "", "NA", "", "FAIL", "Différence maximale de température entre les cellules"], ["DeltaV  (mV)", "", "NA", "", "FAIL", "Différence maximale de tension entre les cellules"]] ("Tableau"), "ligne à traiter"=w367) -> ("result string"=w368:string, "Numout"=w364:i32, "errout"=w369:errorcluster)  [unwired: 10 in]
          }
          frame "Hydrau" {
            w375 = 0 ("index (row)")
            n119 = Index Array(array=w403) -> (element #3=w379:string)  [unwired: 3 in, 2 out]
            n120 = Fract/Exp String To Number(string=w379) -> (number=w378:dbl)  [unwired: 3 in, 1 out]
            n121 = In Range and Coerce(upper limit=w402, x=w378, lower limit=w401) -> (In Range?=w373:bool)  [unwired: 1 out]
            n122 = Build Array(w373) -> (w386:bool[])
            n123 = Increment(x=w400) -> (x+1=w399:i32)
            n124 = call "DataCell_NbPASSFAIL_Bool.vi"("Tableau en entrée"=w386) -> ("Chaîne"=w384:string, "Chaîne 2"=w385:string)  [unwired: 8 in, 1 out]
            n125 = Number To Decimal String(number=w399) -> (decimal integer string=w390:string)  [unwired: 1 in]
            n126 = call <userlib>:"PASSFAIL.vi"("E"=w373) -> ("S"=w377:string)  [unwired: 10 in]
            n127 = Number To Fractional String(number=w402, precision (6)=i16 2) -> (F-format string=w382:string)  [unwired: 2 in]
            n128 = Number To Fractional String(number=w401, precision (6)=i16 2) -> (F-format string=w371:string)  [unwired: 2 in]
            n129 = Build Array(w390, "Continuité Hydrau" ("élément"), w385, w384, "NA" ("élément")) -> (w393:string[])
            n130 = Replace Array Subset(array=string[][] [["Continuité blocs hydrauliques supérieurs  (mOhms)", "", "", "", "", "Vérification de la continuité des blocs hydrauliques supérieurs"]] ("Tableau"), new element #1=w379, index (row) #1=w375, index (col) #1=1 ("disabled index (col)"), new element #2=w382, index (row) #2=w375, index (col) #2=3 ("disabled index (col)"), new element #3=w371, index (row) #3=w375, index (col) #3=2 ("disabled index (col)"), new element #4=w377, index (row) #4=w375, index (col) #4=4 ("disabled index (col)")) -> (w387:string[][])
            n131 = call "HTML_Table_Head.vi"("entrée d'erreur (pas d'erreur)"=w397, "Tableau"=w393, "chaîne en entrée"=w396) -> ("sortie d'erreur"=w392:errorcluster, "result string"=w391:string)  [unwired: 7 in]
            n132 = call "HTML_Table_Data.vi"("entrée d'erreur (pas d'erreur)"=w392, "Tableau"=w387, "chaîne en entrée"=w391) -> ("sortie d'erreur"=w398:errorcluster, "result string"=w395:string)  [unwired: 7 in]
          }
          frame "NULL", Default {
            # "NULL"
          }
        }
      }
    }
  }
  n133 = call "BDDOP300.vi"("errin"=w3, "DATA IN"="BDD") -> ("chaîne concaténée"=→"chaîne concaténée":string)  [unwired: 8 in, 1 out]
  n134 = Search and Replace String(replace all?=TRUE ("tout remplacer ? (F)"), input string=w67, search string="<td class=\"core1 testpass\">FAIL</td>" ("chaîne recherchée"), replace string="<td class=\"core1 testfail\">FAIL</td>" ("chaîne de remplacement (\"\")"), error in=w3) -> (result string=w52:string, number of replacements=w47:i32, error out=w63:errorcluster)  [unwired: 3 in, 1 out]
  n135 = Search and Replace String(replace all?=TRUE ("tout remplacer ? (F)"), input string=w52, search string="<td class=\"core1 testpass\">PASS</td>" ("chaîne recherchée"), error in=w63) -> (number of replacements=w55:i32, error out=w59:errorcluster)  [unwired: 4 in, 2 out]
  "nombre de remplacements" <- w55
  n136 = Number To Decimal String(number=w55) -> (decimal integer string=w54:string)  [unwired: 1 in]
  n137 = Number To Decimal String(number=w47) -> (decimal integer string=w53:string)  [unwired: 1 in]
  n138 = Search and Replace String(input string=w52, search string="<!--NBTESTOK-->" ("chaîne recherchée"), replace string=w54, error in=w59) -> (result string=w60:string, error out=w58:errorcluster)  [unwired: 4 in, 2 out]
  n139 = Equal To 0?(x=w47) -> (x = 0?=w39:bool)
  n140 = Search and Replace String(input string=w60, search string="<!--NBTESTKO-->" ("chaîne recherchée"), replace string=w53, error in=w58) -> (result string=w42:string, error out=w46:errorcluster)  [unwired: 4 in, 2 out]
  n141 = Search and Replace String(input string=w42, search string="Résultat du test :\t</td><td class=\"resume5\" colspan=\"3\"><div><span style=\"float:left\" id=\"result\"><font size = \"5pt\" color=\"green\"><b>CONFORME</b>", replace string="Résultat du test :\t</td><td class=\"resume5\" colspan=\"3\"><div><span style=\"float:left\" id=\"result\"><font  size = \"5pt\" color=\"red\"><b>NON CONFORME</b>", error in=w46) -> (result string=w13:string, error out=w45:errorcluster)  [unwired: 4 in, 2 out]
  n142 = Search and Replace String(input string=w13, search string=".resume1,.resume3,.resume4,.resume5,.resume6,.resume7{background-color:#e6feef;padding:7px;border:1px solid black;}\n.resume0{border:1px solid black;background-color:#e6feef;font-weight: bold;padding:0px;text-align: center;}", replace string=".resume1,.resume3,.resume4,.resume5,.resume6,.resume7{background-color:#fdebd0;padding:7px;border:1px solid black;}\n.resume0{border:1px solid black;background-color:#fdebd0;font-weight: bold;padding:0px;text-align: center;}") -> (result string=w12:string)  [unwired: 5 in, 3 out]
  n143 = Select(t=w42, s=w39, f=w12) -> (s? t:f=w43:string)
  "Chaîne" <- w43
  n144 = Not Equal?(x=w34, y=path "") -> (x != y?=w36:bool)
  n145 = Open/Create/Replace File(file path (use dialog)=w68, error in=w45, operation (0:open)=w51) -> (refnum out=w74:refnum<file>, error out=w76:errorcluster)  [unwired: 3 in, 1 out]
  n146 = case shown="True" w36 {
    tunnel: w51 -> [_ w412]
    tunnel: w34 -> [_ w411]
    tunnel: w45 -> [_ w410]
    tunnel: w43 -> [_ w409]
    tunnel: [errorcluster {"status"=FALSE, "code"=0, "source"=""} ("error out") w408] -> w41
    frame False {
    }
    frame True {
      n147 = Open/Create/Replace File(file path (use dialog)=w411, error in=w410, operation (0:open)=w412) -> (refnum out=w413:refnum<file>, error out=w415:errorcluster)  [unwired: 3 in, 1 out]
      n148 = Write to Text File(file (use dialog)=w413, text=w409, error in=w415) -> (refnum out=w414:refnum<file>, error out=w416:errorcluster)  [unwired: 1 in, 1 out]
      n149 = Close File(refnum=w414, error in=w416) -> (error out=w408:errorcluster)  [unwired: 1 out]
    }
  }
  n150 = Write to Text File(file (use dialog)=w74, text=w43, error in=w76) -> (refnum out=w75:refnum<file>, error out=w77:errorcluster)  [unwired: 1 in, 1 out]
  n151 = Close File(refnum=w75, error in=w77) -> (error out=w40:errorcluster)  [unwired: 1 out]
  n152 = Merge Errors(w40, w41) -> (w38:errorcluster)
  "sortie d'erreur" <- w38
  n153 = Compound Arithmetic op=AND ("Opérateur arithmétique")(w39, invert w38) -> (→"tout bon":bool)
